vi "find key in table.vi"(10 "key":string, 11 "lookup table":T1(array[cluster])) -> (1 "Value Array":dbl[](array[numeric]), 2 "location":i32, 3 "found":bool)   [LabVIEW 2021]
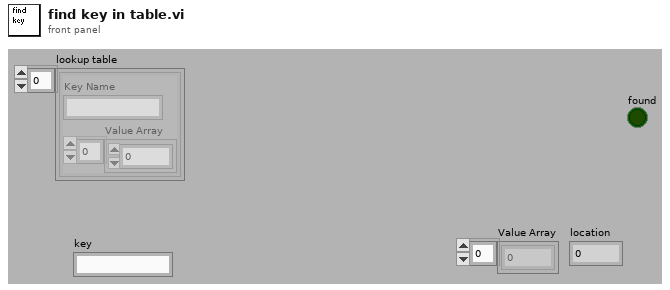
[diagram p1: front panel]
types:
  T1 = cluster{"Key Name":string, "Value Array":dbl[]}[]
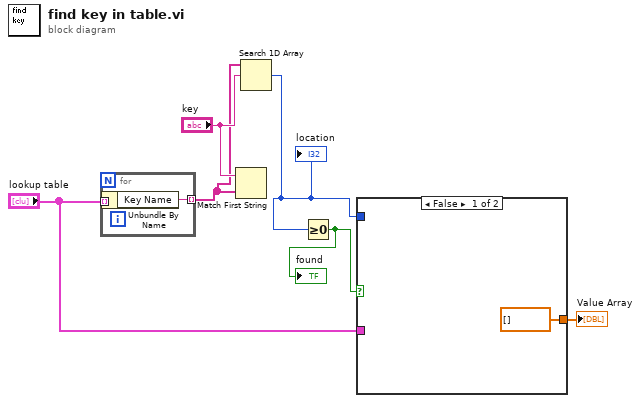
[diagram p0: block diagram]
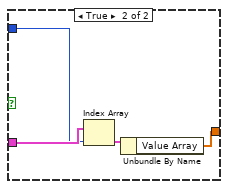
[diagram p2: hidden frame]
diagram:
  n1 = for {
    tunnel: "lookup table" -> [w8] mode=indexing
    tunnel: [w7] -> w2 mode=indexing
    n2 = Unbundle By Name(w8) -> ("Key Name"=w7:string)
  }
  n3 = Match First String(2:w2, 3:"key") -> ()  [unwired: 2 out]
  n4 = Search 1D Array(1D array=w2, element="key") -> (index of element=w1:i32)  [unwired: 1 in]
  "location" <- w1
  n5 = Greater Or Equal To 0?(x=w1) -> (x >= 0?=w5:bool)
  "found" <- w5
  n6 = case shown="False" w5 {
    tunnel: "lookup table" -> [_ w13]
    tunnel: w1 -> [_ w12]
    tunnel: [dbl[] [] ("Value Array") w10] -> w4
    frame False {
    }
    frame True {
      n7 = Index Array(array=w13, index=w12) -> (element=w11:cluster{"Key Name":string, "Value Array":dbl[]})
      n8 = Unbundle By Name(w11) -> ("Value Array"=w10:dbl[])
    }
  }
  "Value Array" <- w4
